vi "subVI_explodeStringArray.vi"(7 "Array":string[](array[string])) -> (6 "x":string, 8 "y":string, 10 "z":string)   [LabVIEW 2013]
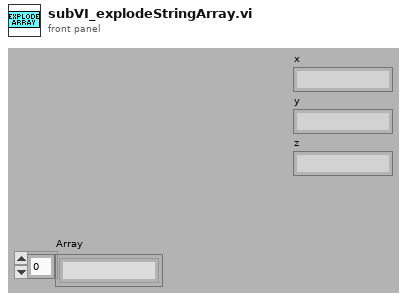
[diagram p1: front panel]
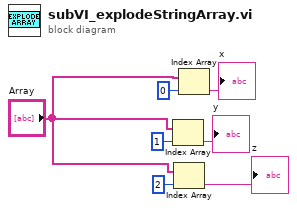
[diagram p0: block diagram]
diagram:
  n1 = Index Array(array="Array", index=1) -> (element=→"y":string)
  n2 = Index Array(array="Array", index=2) -> (element=→"z":string)
  n3 = Index Array(array="Array", index=0) -> (element=→"x":string)
